vi "GetLanguage.vi"(8 "error in (no error)":errorcluster, 11 "FencedCodeBlock in":refnum<class "FencedCodeBlock.lvclass">) -> (0 "error out":errorcluster, 2 "Language":string, 3 "FencedCodeBlock out":refnum<class "FencedCodeBlock.lvclass">)   [LabVIEW 2021, in "LvMarkdown.lvlib" / "FencedCodeBlock.lvclass"]
uses:
  FencedCodeBlock.lvclass
  FencedCodeBlock.lvclass/FencedCodeBlock.ctl
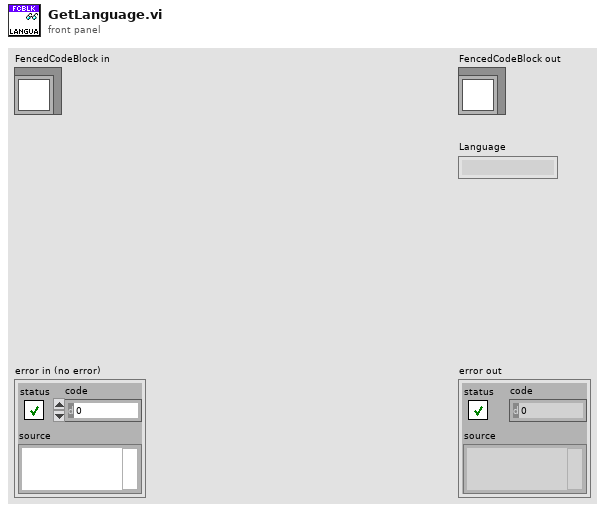
[diagram p1: front panel]
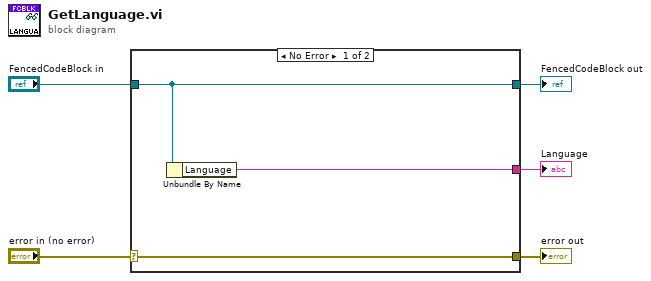
[diagram p0: block diagram]
diagram:
  n1 = case shown="No Error" "error in (no error)" {
    selector: "error in (no error)" -> [w8 w9]
    tunnel: [w8 w9] -> w4
    tunnel: [w7 w10] -> w2
    tunnel: "FencedCodeBlock in" -> [w7 w10]
    tunnel: [w6 _] -> w1
    frame No Error {
      n2 = Unbundle By Name(w7) -> ("Language"=w6:string)
    }
    frame Error {
    }
  }
  "error out" <- w4
  "FencedCodeBlock out" <- w2
  "Language" <- w1
